vi "Configure Trigger Source.vi"(8 "error in (no error)":errorcluster, 9 "External Level":dbl, 10 "Trigger Source":enum16{"Immediate", "External"}(ring), 11 "MXA in":refnum<class "MXA.lvclass">) -> (0 "error out":errorcluster, 3 "MXA out":refnum<class "MXA.lvclass">)   [LabVIEW 2020, in "MXA.lvclass"]
uses:
  MXA.lvclass
  C:/Sandbox/RF Bench/Source Code/WiSpry Test Framework/Instruments/Instrument.lvclass
  Instrument.lvclass/Instrument.ctl
  <instrlib>/Agilent MXA Series/Public/Configure/Trigger/Configure Trigger (Normal).vi
  Instrument.lvclass
  <instrlib>/Agilent MXA Series/Agilent MXA Series.lvlib
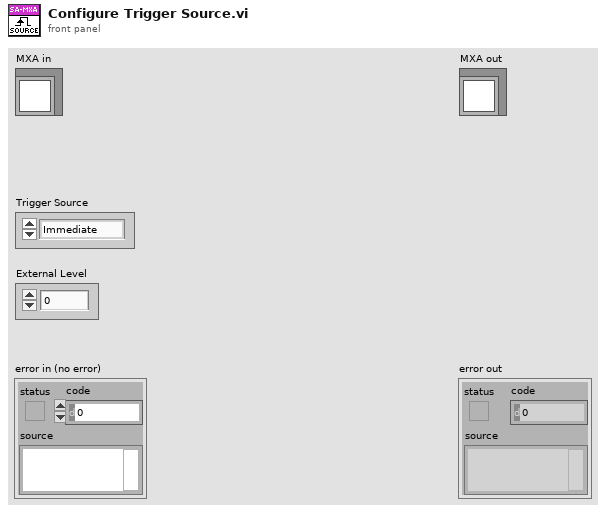
[diagram p1: front panel]
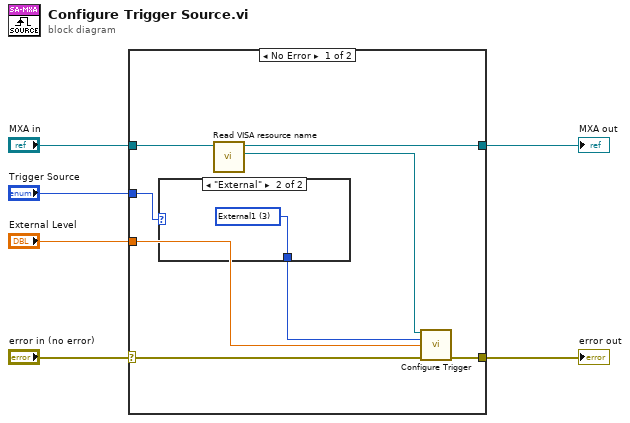
[diagram p0: block diagram]
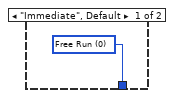
[diagram p2: hidden frame]
diagram:
  n1 = case shown="No Error" "error in (no error)" {
    selector: "error in (no error)" -> [w11 w18]
    tunnel: "MXA in" -> [w14 w17]
    tunnel: [w10 w18] -> w5
    tunnel: [w13 w17] -> w4
    tunnel: "Trigger Source" -> [w9 _]
    tunnel: "External Level" -> [w8 _]
    frame No Error {
      n2 = case shown="\"External\"" w9 {
        tunnel: [w15 w16] -> w7
        frame "Immediate", Default {
          w15 = 0 items=["Free Run", "Video", "Line", "External1", "External2", "RF Burst"] ("Trigger Source (0: Free Run)")
        }
        frame "External" {
          w16 = 3 items=["Free Run", "Video", "Line", "External1", "External2", "RF Burst"] ("Trigger Source (0: Free Run)")
        }
      }
      n3 = call "Read VISA resource name.vi"("Instrument in"=w14) -> ("VISA resource name"=w12:refnum<visa-resource-name>, "Instrument out"=w13:refnum<class "MXA.lvclass">)  [unwired: 9 in]
      n4 = call-poly <instrlib>:"Configure Trigger.vi"("VISA resource name"=w12, "Trigger Source (0: Free Run)"=w7, "Trigger Level (-20 dBm)"=w8, "error in (no error)"=w11) -> ("error out"=w10:errorcluster)  [unwired: 10 in, 1 out]
    }
    frame Error {
    }
  }
  "error out" <- w5
  "MXA out" <- w4
